vi "5-Forebrain.vi"() -> ()   [LabVIEW 2010]
doc: "This VI acts as the MIDbrain in the Olin Robotics Architecture. It interacts with neural clusters on both the Forebrain and Hindbrain as shown in teh respective control panel dynamic documentation diagrams."
uses:
  4-High Neurons/How Sensor Typedef.ctl
  6-OCU Neurons/MainControls.ctl
  6-OCU Neurons/MainIndicators.ctl
  4-High Neurons/4.4-How Sensor Typedef.ctl
  4-High Neurons/4.2-Where Sensor Typedef.ctl
  4-High Neurons/Current GPS Data.ctl
  3-Midbrain/3.2-Where/_typedefs/3.2.1-VectorNav Data.ctl
  5-Forebrain/5.0-Global.vi
panel:
  in  "Tab Control":T1(tab)
  out "5.2.3 Where Am I?  Sensor":T2 {"4.2.2- Current GPS Data"."Longitude (dd.mmmmmm)" format="%#.6g"; "4.2.2- Current GPS Data"."Lattitude (dd.mmmmmm)" format="%#.6g"}
  out "5.3.3 How Am I? Sensor":T5
  out "5.3.1 MissionTimeAuto":dbl(knob) scale=0.0..10.0
  out "5.7.1 AutoModeDatums":T6
  out "5.7.2 Main Indicators":T7
  in  "Stop":bool
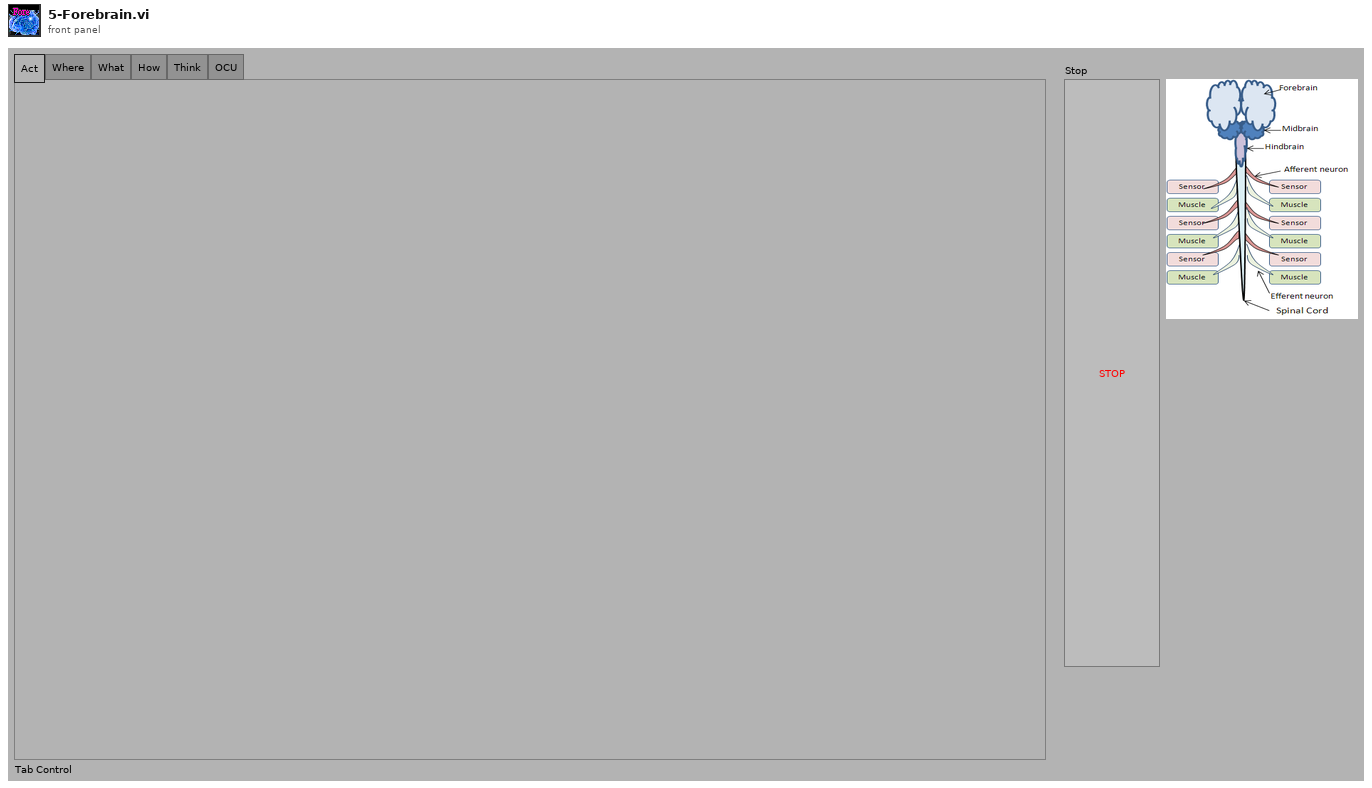
[diagram p1: front panel]
types:
  T1 = enum32{"Act", "Where", "What", "How", "Think", "OCU"}
  T2 = typedef "4.2-Where Sensor Typedef.ctl" = cluster{"4.2.2- Current GPS Data":T3, "4.2.1-VectorNav Data":T4, "4.2.1-VectorNav Status":string}
  T3 = typedef "Current GPS Data.ctl" = cluster{"Lattitude (dd.mmmmmm)":ext, "Longitude (dd.mmmmmm)":ext, "EST Time":timestamp}
  T4 = typedef "3.2.1-VectorNav Data.ctl" = cluster{"Yaw":dbl, "Pitch":dbl, "Roll":dbl}
  T5 = typedef "How Sensor Typedef.ctl" = cluster{"Motor Speed Integer":i32, "Drive Position Integer":i32, "Lidar Position Integer":i32, "Lidar Motor Position Integer":i32, "Steering Position Integer":i32, "Battery Voltage Fxp":dbl, "Drive Encoder Cable Check":bool, "Lidar Drive Encoder Cable Check":bool, "Steer Encoder Cable Check":bool, "Lidar Pos Encoder Cable Check":bool, "Mod Buttons & Blinky Cable Check":bool, "Lidar Data Cable Check":bool, "Drive Motor Cable Check":bool, "Vector Nav Cable Check":bool, "Lidar Drive Cable Check":bool, "Steer Drive Cable Check":bool, "Reverse?":bool, "2.1  Steering Control Voltage":dbl, "2.1 Drive Control Voltage":dbl, "2.1  Lidar Control Voltage":dbl, "2.5.7 A*B":dbl, "2.1  Steering PID Output":dbl, "2.1 Drive PID Output":dbl, "2.1  Lidar PID Output":dbl, "2.1.1 Drive Error":dbl, "2.1.1 Drive Error I":dbl, "2.1.1 Drive Error D":dbl, "2.1.2 Steering Error":dbl, "2.1.2 Steering Error I":dbl, "2.1.2 Steering Error D":dbl, "2.1.3 Lidar Error":dbl, "2.1.3 Lidar Error I":dbl, "2.1.3 Lidar Error D":dbl, "VectorNav Ack Query":bool, "VectorNav Read Byte":u8, "VectorNav Read Status":enum16{"Waiting", "Reading", "Done"}}
  T6 = typedef "MainControls.ctl" = cluster{"RunAutoMode":bool, "Rerun MDF":bool, "Pause":bool}
  T7 = typedef "MainIndicators.ctl" = cluster{"4.4 How Am I? Sensor":T8, "How?":bool, "Where?":bool, "What?":bool}
  T8 = typedef "4.4-How Sensor Typedef.ctl" = cluster{"Motor Speed Integer":i32, "Drive Position Integer":i32, "Lidar Position Integer":i32, "Lidar Motor Position Integer":i32, "Steering Position Integer":i32, "Battery Voltage Fxp":dbl, "Drive Encoder Cable Check":bool, "Lidar Drive Encoder Cable Check":bool, "Steer Encoder Cable Check":bool, "Lidar Pos Encoder Cable Check":bool, "Mod Buttons & Blinky Cable Check":bool, "Lidar Data Cable Check":bool, "Drive Motor Cable Check":bool, "Vector Nav Cable Check":bool, "Lidar Drive Cable Check":bool, "Steer Drive Cable Check":bool, "Reverse?":bool, "2.1  Steering Control Voltage":dbl, "2.1 Drive Control Voltage":dbl, "2.1  Lidar Control Voltage":dbl, "2.5.7 A*B":dbl, "2.1  Steering PID Output":dbl, "2.1 Drive PID Output":dbl, "2.1  Lidar PID Output":dbl, "2.1.1 Drive Error":dbl, "2.1.1 Drive Error I":dbl, "2.1.1 Drive Error D":dbl, "2.1.2 Steering Error":dbl, "2.1.2 Steering Error I":dbl, "2.1.2 Steering Error D":dbl, "2.1.3 Lidar Error":dbl, "2.1.3 Lidar Error I":dbl, "2.1.3 Lidar Error D":dbl, "VectorNav Ack Query":bool, "VectorNav Read Byte":u8, "VectorNav Read Status":enum16{"Waiting", "Reading", "Done"}}
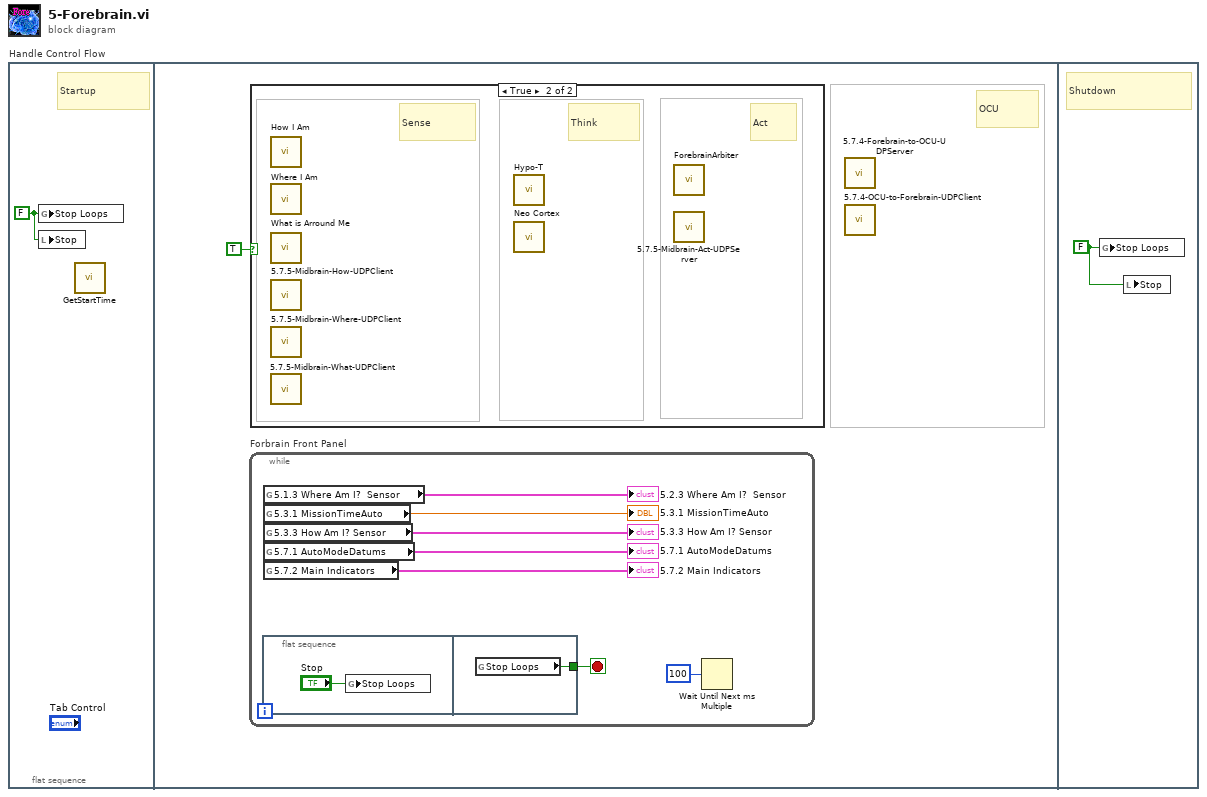
[diagram p0: block diagram]
diagram:
  n1 = flat-sequence "Handle Control Flow" {
    frame #0 {
      w1 = FALSE ("Stop Loops")
      # "Startup"
      n2 = global write "5.0-Global.vi" "Stop Loops"(w1) -> ()
      n3 = local write "Stop"(w1) -> ()
      n4 = call "GetStartTime.vi"() -> ()  [unwired: 12 in]
    }
    frame #1 {
      # "OCU"
      n5 = while "Forbrain Front Panel" {
        stop <- w6 stop-if-true
        n6 = flat-sequence {
          tunnel: [w11] -> w6
          frame #0 {
            n7 = global write "5.0-Global.vi" "Stop Loops"("Stop") -> ()
          }
          frame #1 {
            n8 = global read "5.0-Global.vi" "Stop Loops"() -> (w11:bool)
          }
        }
        n9 = global read "5.0-Global.vi" "5.1.3 Where Am I?  Sensor"() -> (→"5.2.3 Where Am I?  Sensor":T2)
        n10 = global read "5.0-Global.vi" "5.3.1 MissionTimeAuto"() -> (→"5.3.1 MissionTimeAuto":dbl)
        n11 = global read "5.0-Global.vi" "5.3.3 How Am I? Sensor"() -> (→"5.3.3 How Am I? Sensor":T5)
        n12 = global read "5.0-Global.vi" "5.7.1 AutoModeDatums"() -> (→"5.7.1 AutoModeDatums":T6)
        n13 = global read "5.0-Global.vi" "5.7.2 Main Indicators"() -> (→"5.7.2 Main Indicators":T7)
        n14 = Wait Until Next ms Multiple(millisecond multiple=u32 100 ("milliseconds to wait")) -> ()  [unwired: 1 out]
      }
      n15 = case shown="True" TRUE {
        frame False {
        }
        frame True {
          # "Act"
          # "Think"
          # "Sense"
          n16 = call "How I Am.vi"() -> ()  [unwired: 5 in]
          n17 = call "Where I Am.vi"() -> ()  [unwired: 4 in]
          n18 = call "What is Arround Me.vi"() -> ()  [unwired: 3 in, 1 out]
          n19 = call "5.7.5-Midbrain-How-UDPClient.vi"() -> ()  [unwired: 7 in]
          n20 = call "5.7.5-Midbrain-Where-UDPClient.vi"() -> ()  [unwired: 7 in]
          n21 = call "5.7.5-Midbrain-What-UDPClient.vi"() -> ()  [unwired: 7 in]
          n22 = call "Hypo-T.vi"() -> ()  [unwired: 3 in, 1 out]
          n23 = call "Neo Cortex.vi"() -> ()  [unwired: 1 in]
          n24 = call "ForebrainArbiter.vi"() -> ()  [unwired: 15 in, 1 out]
          n25 = call "5.7.5-Midbrain-Act-UDPServer.vi"() -> ()  [unwired: 1 in]
        }
      }
      n26 = call "5.7.4-Forebrain-to-OCU-UDPServer.vi"() -> ()  [unwired: 1 in]
      n27 = call "5.7.4-OCU-to-Forebrain-UDPClient.vi"() -> ()  [unwired: 1 in]
    }
    frame #2 {
      w12 = FALSE ("Stop Loops")
      # "Shutdown"
      n28 = global write "5.0-Global.vi" "Stop Loops"(w12) -> ()
      n29 = local write "Stop"(w12) -> ()
    }
  }
